vi "Load Procedure.vi"(8 "error in (no error)":errorcluster, 10 "Procedure":path=path "Standard Nova Procedures/Cyclic voltammetry.nox", 11 "Instrument":refnum<k24>) -> (0 "error out":errorcluster, 1 "Contains":bool, 2 "Numeric":i32, 3 "LoadProcedure":refnum<k24>)   [LabVIEW 2011]
doc: "Load procedure and checks if the procedure can be executed. The check uses a blacklist xml file. (advanced version)."
uses:
  C:/Program Files/Metrohm Autolab/Autolab SDK 1.10/EcoChemie.Autolab.Sdk.dll
  EcoChemie.Autolab.Sdk.dll
panel:
  in  "Blacklist":path=path "BlackList.xml"
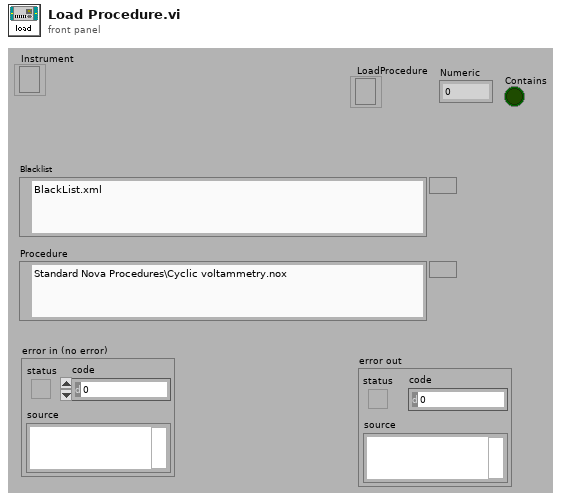
[diagram p1: front panel]
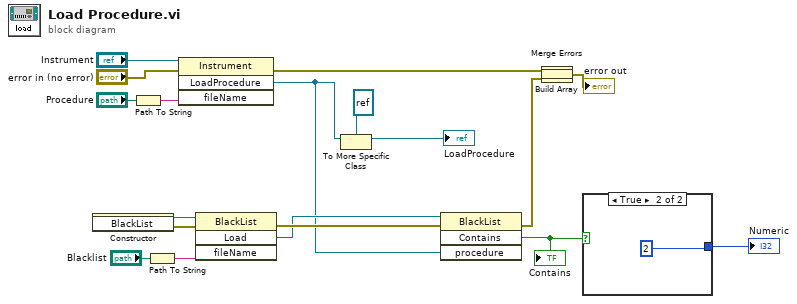
[diagram p0: block diagram]
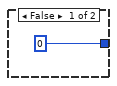
[diagram p2: hidden frame]
diagram:
  n1 = constructor class="BlackList"() -> (reference out=w15:refnum<k24>, error out=w14:errorcluster)  [unwired: 3 in, 1 out]
  n2 = Path To String(path="Procedure") -> (string=w18:string)
  n3 = Path To String(path="Blacklist") -> (string=w5:string)
  n4 = invoke class="Instrument" method="LoadProcedure"(reference="Instrument", error in="error in (no error)", "fileName"=w18) -> (error out=w8:errorcluster, "LoadProcedure"=w2:refnum<k24>)  [unwired: 1 in, 2 out]
  n5 = invoke class="BlackList" method="Load"(reference=w15, error in=w14, "fileName"=w5) -> (error out=w13:errorcluster, "Load"=w12:refnum<k24>)  [unwired: 1 in, 2 out]
  n6 = To More Specific Class(target class=refnum<k24> refnum, reference=w2) -> (specific class reference=→"LoadProcedure":refnum<k24>)  [unwired: 1 in, 1 out]
  n7 = invoke class="BlackList" method="Contains"(reference=w12, error in=w13, "procedure"=w2) -> (error out=w7:errorcluster, "Contains"=w11:bool)  [unwired: 1 in, 2 out]
  "Contains" <- w11
  n8 = Build Array(w8, w7) -> (w1:errorcluster[])
  n9 = Merge Errors(w1) -> (→"error out":errorcluster)
  n10 = case shown="True" w11 {
    tunnel: [0 2] -> w10
    frame False {
    }
    frame True {
    }
  }
  "Numeric" <- w10
